vi "WiFi Serial Println IP.vi"() -> ()   [LabVIEW 2014]
uses:
  <vilib>/LabVIEW Universal Transcriptor/ESP8266 WiFi Wrapper/ESP8266 WiFi Wrapper.lvlib
panel:
  in  "WiFi Mode":T1(ring)=enum."WIFI_AP_STA"
  out "Error Out":errorcluster
  in  "Error In":errorcluster
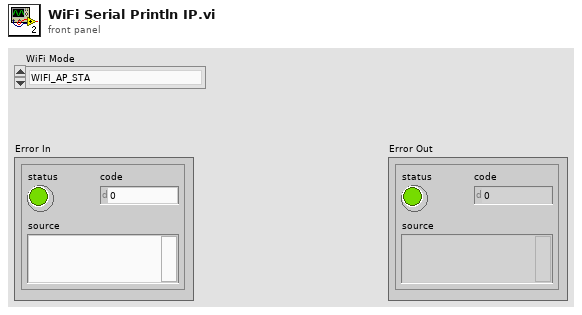
[diagram p1: front panel]
types:
  T1 = enum16{"WIFI_OFF", "WIFI_STA", "WIFI_AP", "WIFI_AP_STA"}
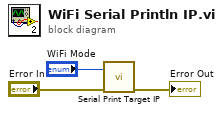
[diagram p0: block diagram]
diagram:
  n1 = call <vilib>:"Serial Print Target IP.vi"("WiFi Mode"="WiFi Mode", "Error In"="Error In") -> ("Error Out"=→"Error Out":errorcluster)  [unwired: 9 in]
